vi "周期设置_CODMn.vi"() -> ()   [LabVIEW 2016, in "斯坦道CODMn.lvlib"]
uses:
  <vilib>/Utility/miscctls.llb/LVPointTypeDef.ctl
  <vilib>/Utility/config.llb/NI_LVConfig.lvlib
panel:
  in  "运行周期":T1={"运行模式"=enum."维护模式", "质控频次"=enum."关闭", "空白核查时间"=2, "跨度核查时间"=6, "24H周期设置"=[]} {"跨度核查时间" items=["00H", "01H", "02H", "03H", "04H", "05H", "06H", "07H", "08H", "09H", "10H", "11H", "12H", "13H", "14H", "15H", "16H", "17H", "18H", "19H", "20H", "21H", "22H", "23H", "关闭"]; "空白核查时间" items=["00H", "01H", "02H", "03H", "04H", "05H", "06H", "07H", "08H", "09H", "10H", "11H", "12H", "13H", "14H", "15H", "16H", "17H", "18H", "19H", "20H", "21H", "22H", "23H", "关闭"]}
  # "运行模式："
  # "质控频次："
  # "空白核查时间："
  # "跨度核查时间："
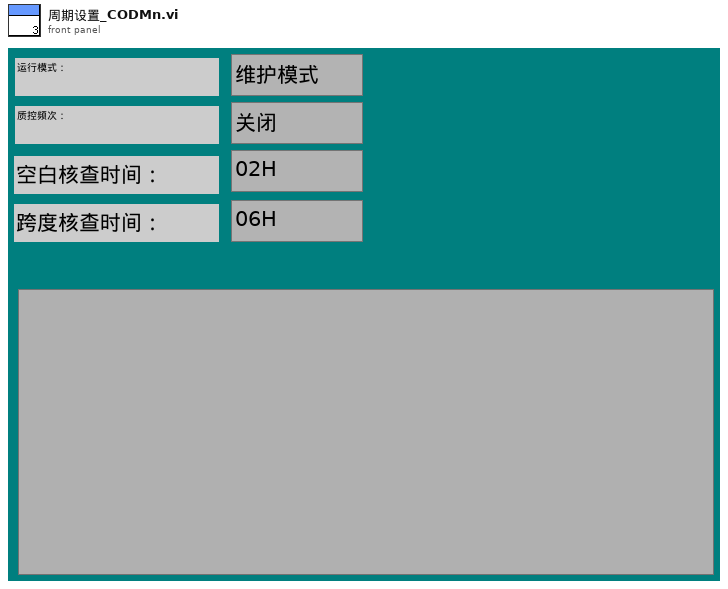
[diagram p1: front panel]
types:
  T1 = cluster{"运行模式":enum16{"维护模式", "常规模式", "应急模式", "质控模式"}, "质控频次":enum16{"关闭", "每天", "星期一", "星期二", "星期三", "星期四", "星期五", "星期六", "星期日"}, "空白核查时间":u16, "跨度核查时间":u16, "24H周期设置":bool[]}
  T2 = typedef "LVPointTypeDef.ctl" = cluster{"Horizontal":i16, "Vertical":i16}
  T3 = cluster{"测量模式":enum16{"水样测量", "标样核查", "零点核查", "跨度核查", "空白测试", "加标回收", "平行样", "校零", "校标"}}
  T4 = enum16{"关闭", "每天", "星期一", "星期二", "星期三", "星期四", "星期五", "星期六", "星期日"}
  T5 = typedef "LVDateTimeRec.ctl" = cluster{"秒数的小数部分":dbl, "秒":i32, "分":i32, "时":i32, "日":i32, "月":i32, "年":i32, "天数（周）":i32, "天数（年）":i32, "DST":i32}
  T6 = typedef "NI_LVConfig.lvlib/Config Data RefNum.ctl" = refnum<k1>
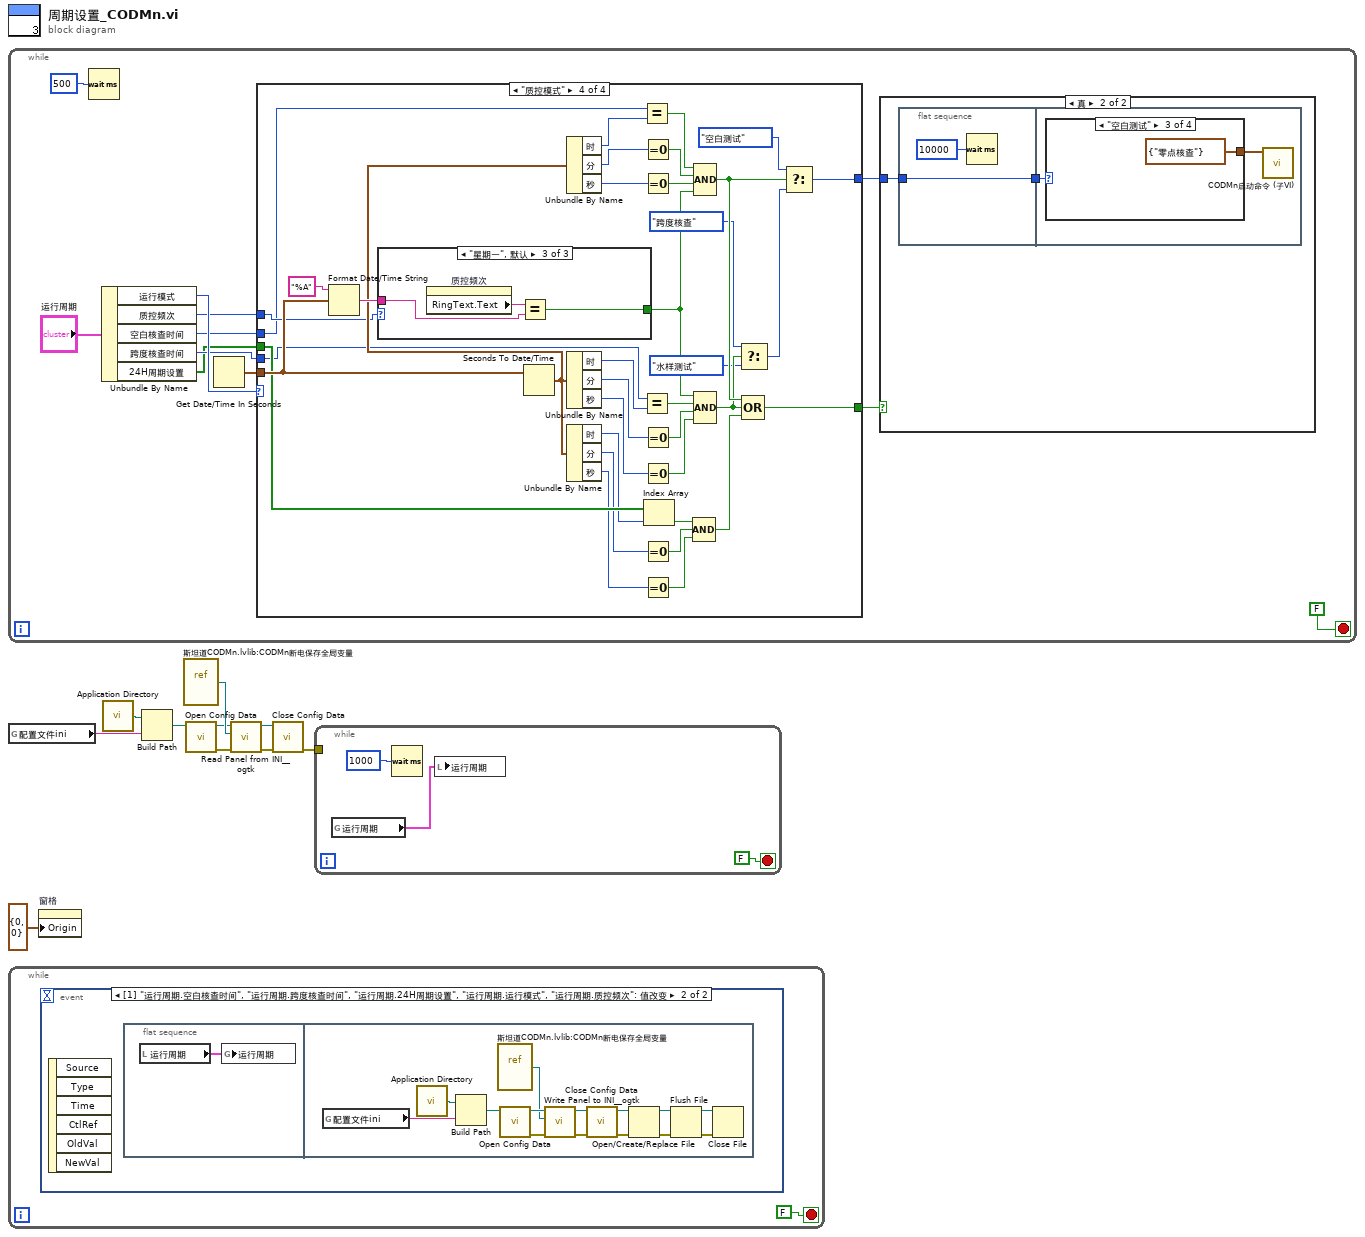
[diagram p0: block diagram]
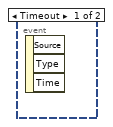
[diagram p2: hidden frame]
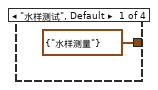
[diagram p4: hidden frame]
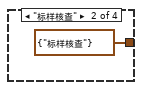
[diagram p5: hidden frame]
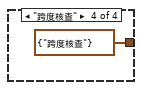
[diagram p6: hidden frame]
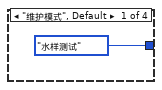
[diagram p7: hidden frame]
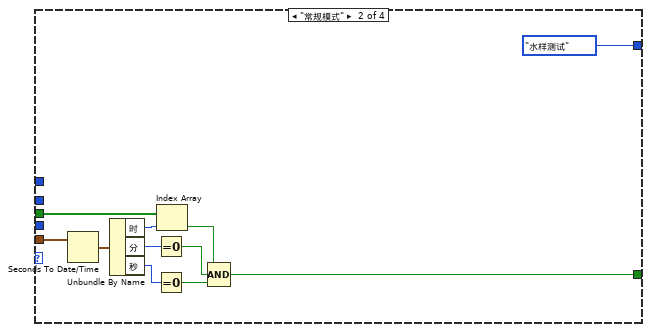
[diagram p8: hidden frame]
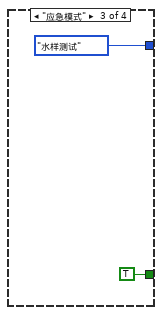
[diagram p9: hidden frame]
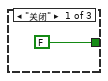
[diagram p10: hidden frame]
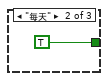
[diagram p11: hidden frame]
diagram:
  n1 = while {
    stop <- FALSE stop-if-true
    n2 = Wait (ms)(milliseconds to wait=u32 500 ("等待时间（毫秒）")) -> ()  [unwired: 1 out]
    n3 = Unbundle By Name("运行周期") -> ("运行模式"=w17:enum16{"维护模式", "常规模式", "应急模式", "质控模式"}, "质控频次"=w16:T4, "空白核查时间"=w15:u16, "跨度核查时间"=w14:u16, "24H周期设置"=w13:bool[])
    n4 = Get Date/Time In Seconds() -> (seconds since 1Jan1904=w21:timestamp)
    n5 = case shown="\"质控模式\"" w17 {
      tunnel: w21 -> [_ w42 _ w81]
      tunnel: w13 -> [_ w39 _ w78]
      tunnel: [_ w33 TRUE w58] -> w12
      tunnel: [enum16{"水样测试", "标样核查", "空白测试", "跨度核查"}."水样测试" ("仪器测试类型") enum16{"水样测试", "标样核查", "空白测试", "跨度核查"}."水样测试" ("仪器测试类型") enum16{"水样测试", "标样核查", "空白测试", "跨度核查"}."水样测试" ("仪器测试类型") w51] -> w11
      tunnel: w16 -> [_ _ _ w48]
      tunnel: w15 -> [_ _ _ w47]
      tunnel: w14 -> [_ _ _ w46]
      frame "维护模式", Default {
      }
      frame "常规模式" {
        n6 = Seconds To Date/Time(time stamp (now)=w42) -> (date time rec=w41:T5)  [unwired: 1 in]
        n7 = Unbundle By Name(w41) -> ("时"=w40:i32, "分"=w38:i32, "秒"=w37:i32)
        n8 = Equal To 0?(x=w38) -> (x = 0?=w35:bool)
        n9 = Equal To 0?(x=w37) -> (x = 0?=w34:bool)
        n10 = Index Array(array=w39, index=w40) -> (element=w36:bool)
        n11 = Compound Arithmetic op=AND ("复合运算")(w36, w35, w34) -> (w33:bool)
      }
      frame "应急模式" {
      }
      frame "质控模式" {
        n12 = Format Date/Time String(time format string (%c)="%A" ("时间格式字符串(%c)"), seconds (now)=w81) -> (date/time string=w79:string)  [unwired: 1 in]
        n13 = case shown="\"星期一\", 默认" w48 {
          tunnel: w79 -> [_ _ w85]
          tunnel: [FALSE TRUE w84] -> w49
          frame "关闭" {
          }
          frame "每天" {
          }
          frame "星期一", Default {
            n14 = property on="质控频次" class="Enum (严格)"() -> ("RingText.Text"=w86:string)  [unwired: 2 in, 2 out]
            n15 = Equal?(x=w86, y=w85) -> (x = y?=w84:bool)
          }
        }
        n16 = Seconds To Date/Time(time stamp (now)=w81) -> (date time rec=w62:T5)  [unwired: 1 in]
        n17 = Unbundle By Name(w62) -> ("时"=w71:i32, "分"=w70:i32, "秒"=w69:i32)
        n18 = Unbundle By Name(w62) -> ("时"=w63:i32, "分"=w64:i32, "秒"=w65:i32)
        n19 = Unbundle By Name(w62) -> ("时"=w77:i32, "分"=w75:i32, "秒"=w73:i32)
        n20 = Equal?(x=w47, y=w71) -> (x = y?=w68:bool)
        n21 = Equal?(x=w46, y=w63) -> (x = y?=w61:bool)
        n22 = Equal To 0?(x=w70) -> (x = 0?=w67:bool)
        n23 = Equal To 0?(x=w69) -> (x = 0?=w66:bool)
        n24 = Equal To 0?(x=w64) -> (x = 0?=w60:bool)
        n25 = Equal To 0?(x=w65) -> (x = 0?=w59:bool)
        n26 = Equal To 0?(x=w75) -> (x = 0?=w74:bool)
        n27 = Equal To 0?(x=w73) -> (x = 0?=w72:bool)
        n28 = Index Array(array=w78, index=w77) -> (element=w76:bool)
        n29 = Compound Arithmetic op=AND ("复合运算")(w76, w74, w72) -> (w50:bool)
        n30 = Compound Arithmetic op=AND ("复合运算")(w68, w67, w66, w49) -> (w57:bool)
        n31 = Compound Arithmetic op=AND ("复合运算")(w49, w61, w60, w59) -> (w55:bool)
        n32 = Select(t=enum16{"水样测试", "标样核查", "空白测试", "跨度核查"}."跨度核查" ("仪器测试类型"), s=w55, f=enum16{"水样测试", "标样核查", "空白测试", "跨度核查"}."水样测试" ("仪器测试类型")) -> (s? t:f=w53:enum16{"水样测试", "标样核查", "空白测试", "跨度核查"})
        n33 = Compound Arithmetic op=OR ("复合运算")(w57, w55, w50) -> (w58:bool)
        n34 = Select(t=enum16{"水样测试", "标样核查", "空白测试", "跨度核查"}."空白测试" ("仪器测试类型"), s=w57, f=w53) -> (s? t:f=w51:enum16{"水样测试", "标样核查", "空白测试", "跨度核查"})
      }
    }
    n35 = case shown="真" w12 {
      tunnel: w11 -> [_ w23]
      frame False {
      }
      frame True {
        n36 = flat-sequence {
          tunnel: w23 -> [w25]
          tunnel: [w25] -> w22
          tunnel: w22 -> [w27]
          frame #0 {
            n37 = Wait (ms)(milliseconds to wait=u32 10000 ("等待时间（毫秒）")) -> ()  [unwired: 1 out]
          }
          frame #1 {
            n38 = case shown="\"空白测试\"" w27 {
              tunnel: [T3 {"测量模式"=enum."水样测量"} ("启动测量模式") T3 {"测量模式"=enum."标样核查"} ("启动测量模式") T3 {"测量模式"=enum."零点核查"} ("启动测量模式") T3 {"测量模式"=enum."跨度核查"} ("启动测量模式")] -> w26
              frame "水样测试", Default {
              }
              frame "标样核查" {
              }
              frame "空白测试" {
              }
              frame "跨度核查" {
              }
            }
            n39 = call "CODMn启动命令 (子VI).vi"("启动测量模式"=w26) -> ()  [unwired: 11 in]
          }
        }
      }
    }
  }
  n40 = global read "COD内部交互全局.vi" "配置文件ini"() -> (w1:string)
  n41 = while {
    stop <- FALSE stop-if-true
    n42 = event shown="[1] \"运行周期.空白核查时间\", \"运行周期.跨度核查时间\", \"运行周期.24H周期设置\", \"运行周期.运行模式\", \"运行周期.质控频次\": 值改变" {
      selector: _ -> [_ _]
      dyn-events: _ -> [_ _]
      timeout: _ -> [_ _]
      event Timeout {
        n43 = event-data() -> ()  [unwired: 1 in, 3 out]
      }
      event "运行周期.空白核查时间", "运行周期.跨度核查时间", "运行周期.24H周期设置", "运行周期.运行模式", "运行周期.质控频次": Value Change {
        n44 = event-data() -> ()  [unwired: 1 in, 6 out]
        n45 = flat-sequence {
          frame #0 {
            n46 = local read "运行周期"() -> (w88:T1)
            n47 = global write "CODMn断电保存全局变量.vi" "运行周期"(w88) -> ()
          }
          frame #1 {
            n48 = global read "COD内部交互全局.vi" "配置文件ini"() -> (w89:string)
            n49 = call <vilib>:"Application Directory.vi"() -> ("Application Directory"=w102:path)
            n50 = Build Path(base path=w102, name or relative path=w89) -> (appended path=w101:path)
            n51 = vi-ref "斯坦道CODMn.lvlib:CODMn断电保存全局变量.vi"() -> (w99:refnum<vi>)
            n52 = call <vilib>:"Open Config Data.vi"("configuration file path"=w101) -> ("error out"=w97:errorcluster, "refnum"=w100:T6)  [unwired: 8 in, 1 out]
            n53 = call <userlib>:"Write Panel to INI__ogtk.vi"("error in (no error)"=w97, "VI ref"=w99, "refnum"=w100) -> ("error out"=w96:errorcluster, "refnum out"=w98:T6)  [unwired: 7 in]
            n54 = call <vilib>:"Close Config Data.vi"("error in (no error)"=w96, "refnum"=w98) -> ("error out"=w91:errorcluster, "file path"=w90:path)  [unwired: 8 in]
            n55 = Open/Create/Replace File(file path (use dialog)=w90, error in=w91) -> (refnum out=w94:refnum<file>, error out=w95:errorcluster)  [unwired: 4 in, 1 out]
            n56 = Flush File(refnum=w94, error in=w95) -> (refnum out=w93:refnum<file>, error out=w92:errorcluster)
            n57 = Close File(refnum=w93, error in=w92) -> ()  [unwired: 2 out]
          }
        }
      }
    }
  }
  n58 = property on="窗格" class="Pane"("Origin"=T2 {"Horizontal"=0, "Vertical"=0} ("原点")) -> ()  [unwired: 2 in, 2 out]
  n59 = call <vilib>:"Application Directory.vi"() -> ("Application Directory"=w4:path)
  n60 = Build Path(base path=w4, name or relative path=w1) -> (appended path=w5:path)
  n61 = vi-ref "斯坦道CODMn.lvlib:CODMn断电保存全局变量.vi"() -> (w7:refnum<vi>)
  n62 = call <vilib>:"Open Config Data.vi"("configuration file path"=w5) -> ("error out"=w9:errorcluster, "refnum"=w6:T6)  [unwired: 8 in, 1 out]
  n63 = call <userlib>:"Read Panel from INI__ogtk.vi"("error in (no error)"=w9, "VI ref"=w7, "refnum"=w6) -> ("error out"=w10:errorcluster, "refnum out"=w8:T6)  [unwired: 7 in]
  n64 = call <vilib>:"Close Config Data.vi"("error in (no error)"=w10, "refnum"=w8) -> ("error out"=w3:errorcluster)  [unwired: 8 in, 1 out]
  n65 = while {
    tunnel: w3 -> [_]
    stop <- FALSE stop-if-true
    n66 = global read "CODMn断电保存全局变量.vi" "运行周期"() -> (w103:T1)
    n67 = Wait (ms)(milliseconds to wait=u32 1000 ("等待时间（毫秒）")) -> ()  [unwired: 1 out]
    n68 = local write "运行周期"(w103) -> ()
  }
